vi "Consumer.vi"(8 "error in (no error)":errorcluster, 9 "Data":variant, 10 "Case ID":string, 11 "Kasli Wrapper in":refnum<class "Kasli Wrapper 2.0.lvclass">) -> (0 "error out":errorcluster, 3 "Kasli Wrapper out":refnum<class "Kasli Wrapper 2.0.lvclass">)   [LabVIEW 2020, in "Kasli Wrapper 2.0.lvlib" / "Kasli Wrapper 2.0.lvclass"]
uses:
  Kasli Wrapper 2.0.lvclass
  C:/Users/marco/Documents/GitHub_Lab/TALOS/talos/Ancestor/Ancestor/Ancestor.lvclass
  C:/Users/marco/Documents/GitHub_Lab/TALOS/talos/Father of all uServices/Father of all uServices/Father of all uServices.lvclass
  Kasli Wrapper 2.0 Consumer Case Selector.ctl
  Ancestor/Ancestor/Ancestor.lvclass/Ancestor.ctl
  Father of all uServices/Father of all uServices/Father of all uServices.lvclass/Father of all uServices.ctl
  Run Utilities/TypeDefs/Messages/Submit Message.ctl
  Run Utilities/TypeDefs/DAQ Control.ctl
  Run Utilities/Run Instance/Run Instance.lvclass
  Father of all uServices/Father of all uServices Messages/Consumer Msg/Consumer Msg.lvclass/Consumer Msg.ctl
  Kasli Wrapper 2.0.lvclass/Kasli Wrapper 2.0.ctl
  Std Selector.ctl
  Guardian/Guardian Messages/Message to uService Msg/Message to uService Msg.lvclass/Message to uService Msg.ctl
  Guardian/Guardian/Requests.ctl
  Guardian/Guardian Messages/Requests from uServices Msg/Requests from uServices Msg.lvclass/Requests from uServices Msg.ctl
  Classes/Log/Log.lvclass/Log.ctl
  Ancestor/Ancestor/Read ID.vi
  Guardian/Guardian Messages/Requests from uServices Msg/Send Requests from uServices.vi
  Guardian/Guardian Messages/Message to uService Msg/Send Message to uService.vi
  Classes/Log/Write.vi
  FGV/Error Memory/Get Error Description.vi
  Support VIs/Get PC name.vi
  Support VIs/Get Class Name.vi
  Support VIs/Date n Time.vi
  FGV/Error Memory/Error Memory Core.vi
  <vilib>/AdvancedString/Delimited String to 1D String Array.vi
  Support VIs/Circus Root Path.vi
  FGV/Error Memory/Error Crt Lvl checker.vi
  FGV/Error Memory/Error Memory Core.vi/40c8088d-b597-4017-91af-faa98e00292e.vi
  FGV/Error Memory/Error Memory Core.vi/d4a3ab98-063c-4e44-b43d-fbdcfe6c2be2.vi
  Father of all uServices/Father of all uServices/Father of all uServices.lvclass
  C:/Users/marco/Documents/GitHub_Lab/TALOS/builds/Actor Framework PPL/Actor Framework.lvlibp/1abvi3w/vi.lib/ActorFramework/Actor/Actor.lvclass
  Support VIs/Global Memory.vi
  <vilib>/Utility/LVClass/Get LV Class Name.vi
  Support VIs/Is in Packed Library.vi
  Support VIs/TALOS Root path.vi
  Support VIs/Read CSV worksheet.vi
  Support VIs/Global Constants.vi
  <vilib>/Utility/error.llb/General Error Handler.vi
  Support VIs/Error Log.vi
  builds/Actor Framework PPL/Actor Framework.lvlibp/1abvi3w/vi.lib/ActorFramework/Actor/Read Self Enqueuer.vi
  <userlib>/_OpenG.lib/lvdata/lvdata.llb/Get Strings from Enum__ogtk.vi
  builds/Actor Framework PPL/Actor Framework.lvlibp/1abvi3w/vi.lib/ActorFramework/Message Enqueuer/Enqueue.vi
  Father of all uServices/Father of all uServices/Children Methods/Get GUI Item Value - String.vi
  Father of all uServices/Father of all uServices/Multiline string updater.vi
  builds/Actor Framework PPL/Actor Framework.lvlibp/1abvi3w/vi.lib/ActorFramework/Actor/Read Caller Enqueuer.vi
  Classes/Log/Rotate.vi
  Ancestor/Ancestor/Ancestor.lvclass
  <vilib>/Comparison/Equal/Equal Functor/Equal Functor.lvclass
  Father of all uServices/Father of all uServices Messages/Consumer Msg/Consumer Msg.lvclass
  <vilib>/regexp/Match Regular Expression.xnode
  Guardian/Guardian Messages/Requests from uServices Msg/Requests from uServices Msg.lvclass
  Guardian/Guardian Messages/Message to uService Msg/Message to uService Msg.lvclass
  Run Utilities/Run Utilities.lvlib
  TALOS.lvlib
  Classes/Log/Log.lvclass
  Guardian/Guardian/Guardian.lvclass
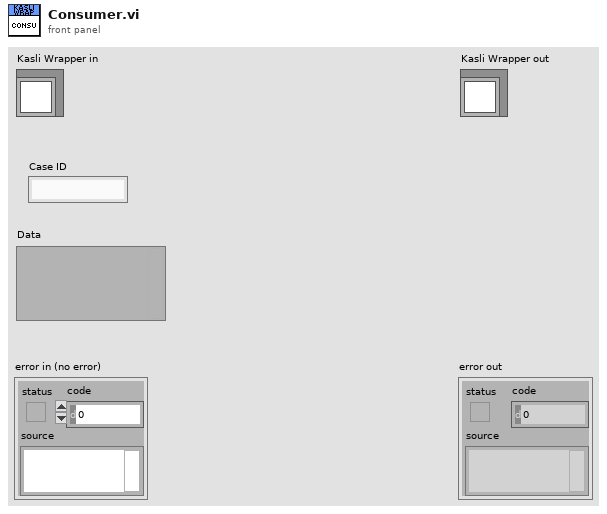
[diagram p1: front panel]
types:
  T1 = typedef "Kasli Wrapper 2.0.lvlib/Kasli Wrapper 2.0.lvclass/Kasli Wrapper 2.0 Consumer Case Selector.ctl" = enum16{"Init", "Submit Script", "Restart Master", "Master StdOut", "Master StdErr", "Client StdOut", "Client StdErr", "Start Logging", "Stop Logging", "Terminate Script", "Close", "Master ProcessExit"}
  T2 = cluster{"Font Name:":string, "Size":i16, "Strikeout?":bool, "Italic?":bool, "Underline?":bool, "Outline?":bool, "Shadow?":bool, "Bold?":bool}
  T3 = enum16{"User-specified Font", "Application Font", "System Font", "Dialog Font"}
  T4 = typedef "TALOS.lvlib/Run Utilities.lvlib/Submit Message.ctl" = cluster{"DAQ Control":T5, "Run Instance":refnum<class "Run Instance.lvclass">}
  T5 = typedef "TALOS.lvlib/Run Utilities.lvlib/DAQ Control.ctl" = enum16{"On", "Off", "External"}
  T6 = typedef "Kasli Wrapper 2.0.lvlib/Kasli Wrapper 2.0.lvclass/Std Selector.ctl" = enum16{"StdOut", "StdErr"}
  T7 = typedef "TALOS.lvlib/Guardian.lvlib/Guardian.lvclass/Requests.ctl" = enum16{"Ready to Launch", "Start RUN", "Stop RUN", "Update DAQ Params", "Update Error Listbox", "Update Run Status", "Update Kasli Log", "Run Stopped with Errors", "Switch uS View"}
  T8 = cluster{"left":i16, "top":i16, "right":i16, "bottom":i16}
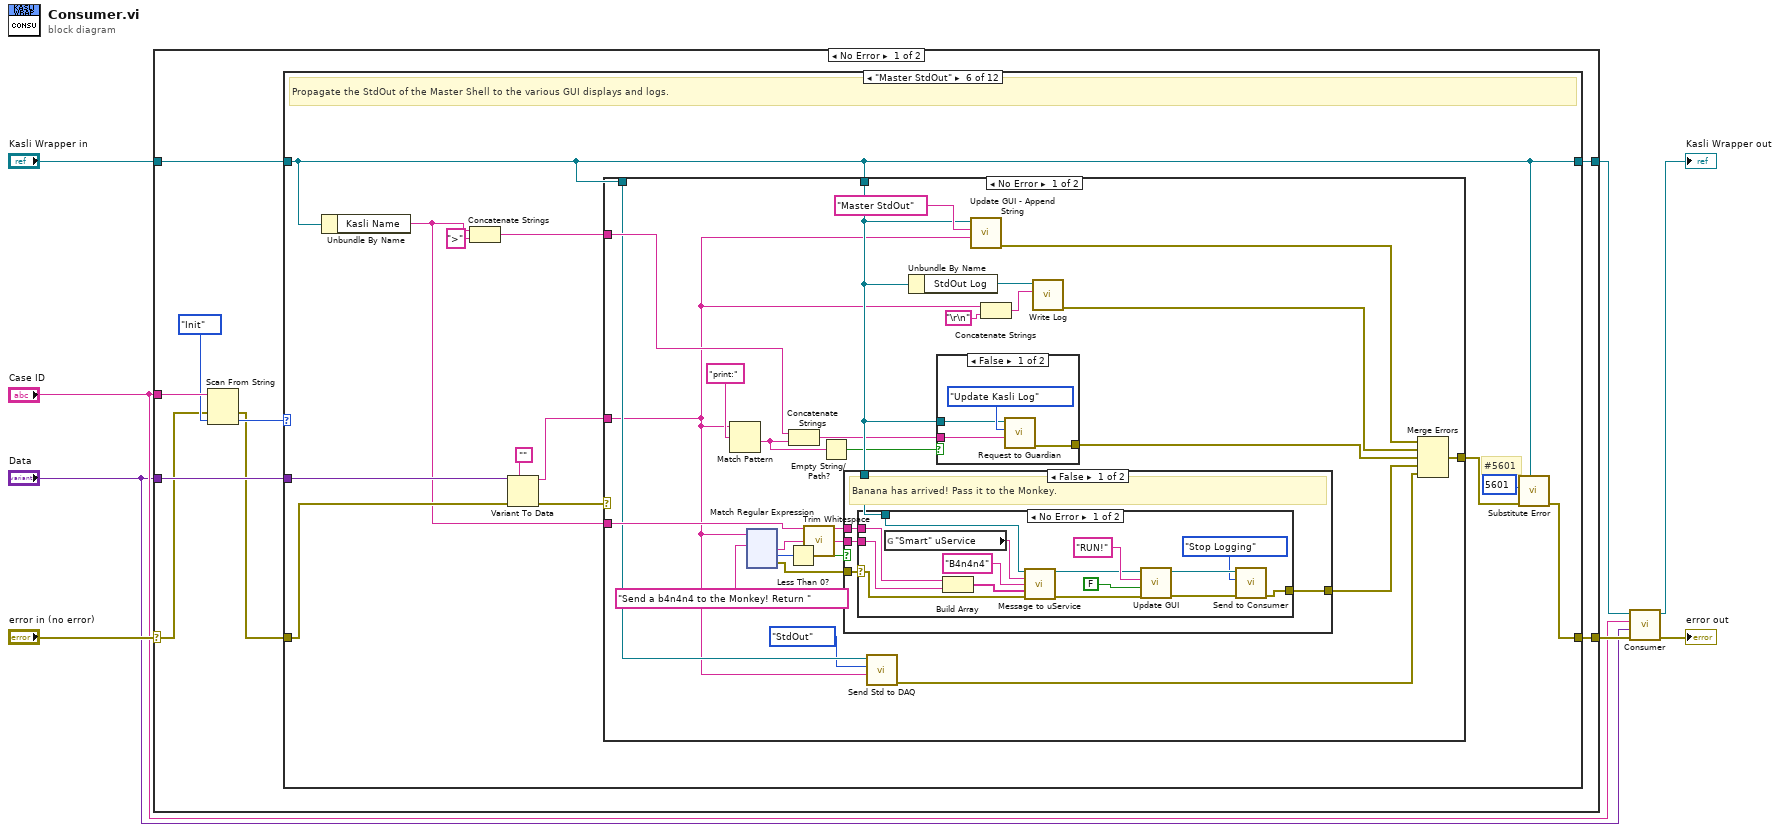
[diagram p0: block diagram]
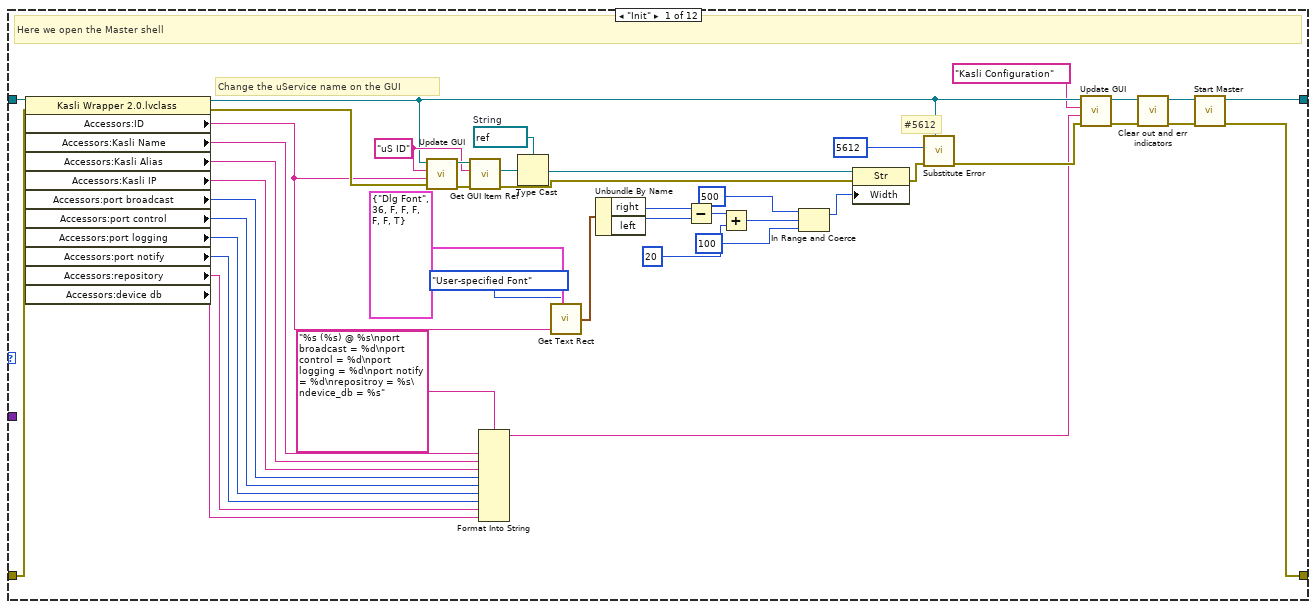
[diagram p2: hidden frame]
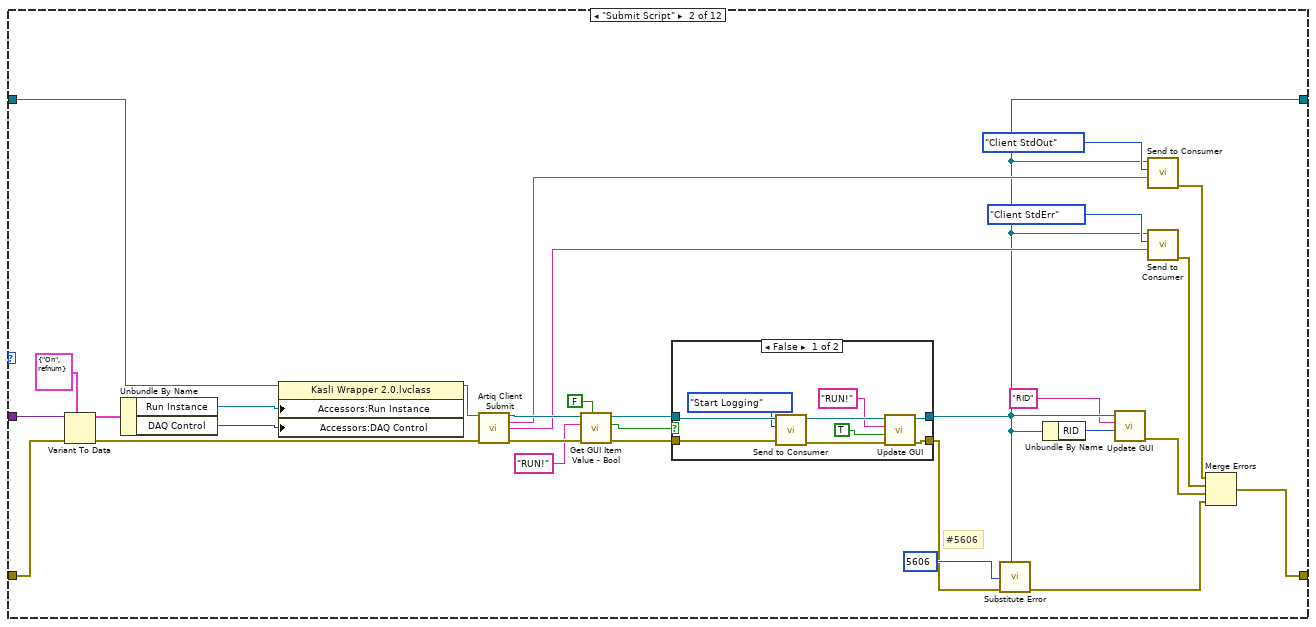
[diagram p3: hidden frame]
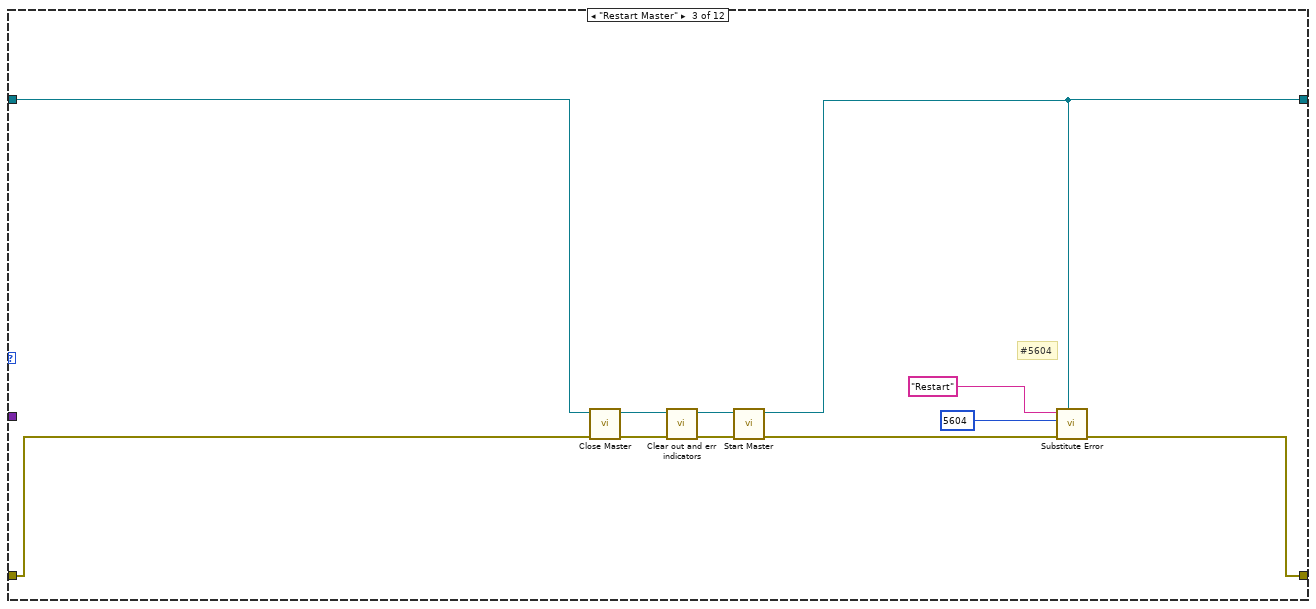
[diagram p5: hidden frame]
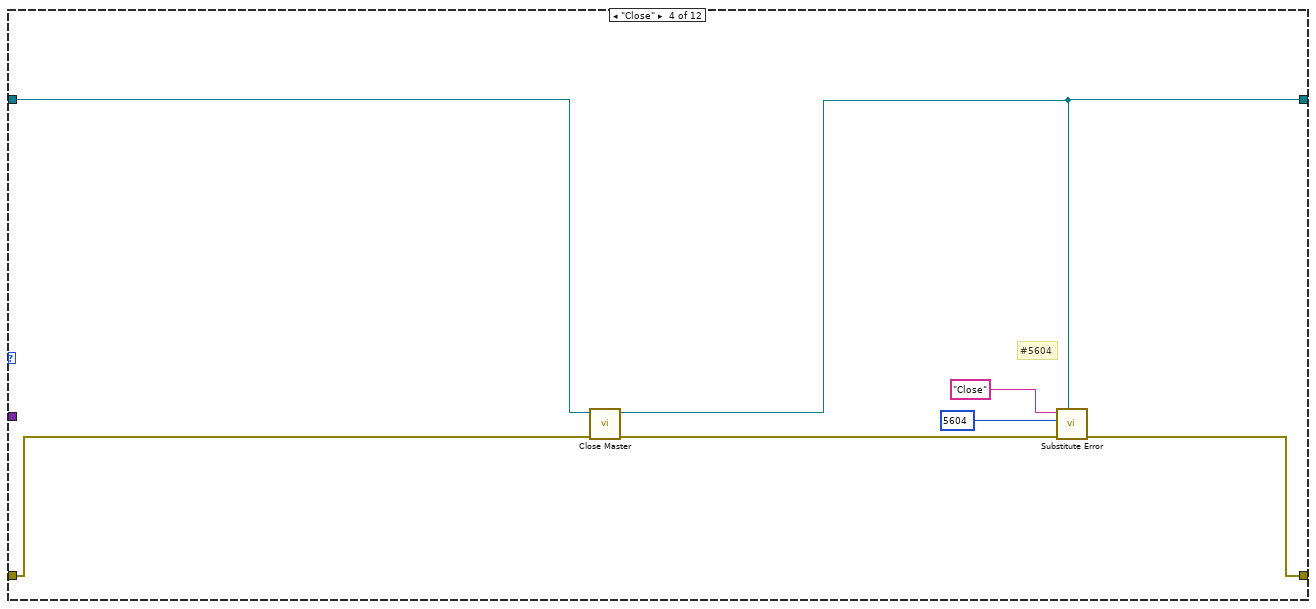
[diagram p6: hidden frame]
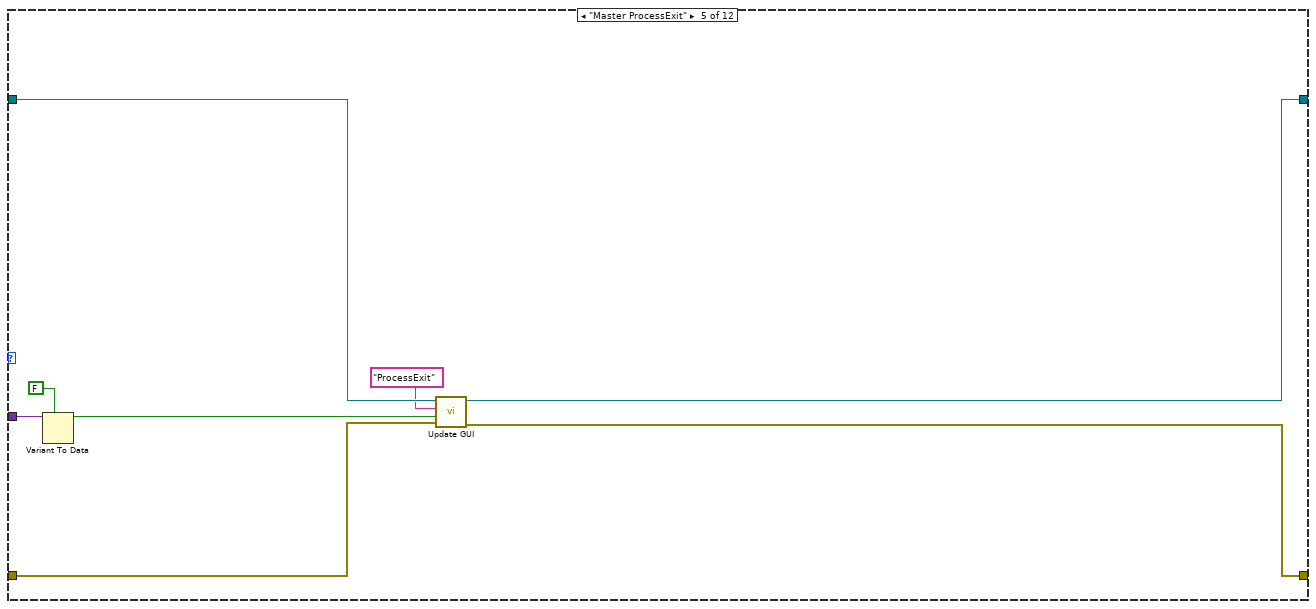
[diagram p7: hidden frame]
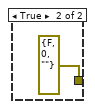
[diagram p8: hidden frame]
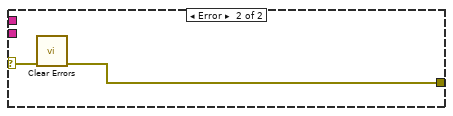
[diagram p9: hidden frame]
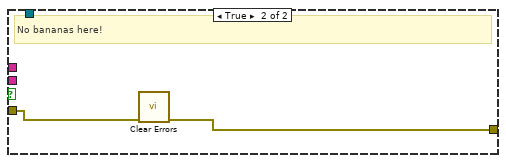
[diagram p10: hidden frame]
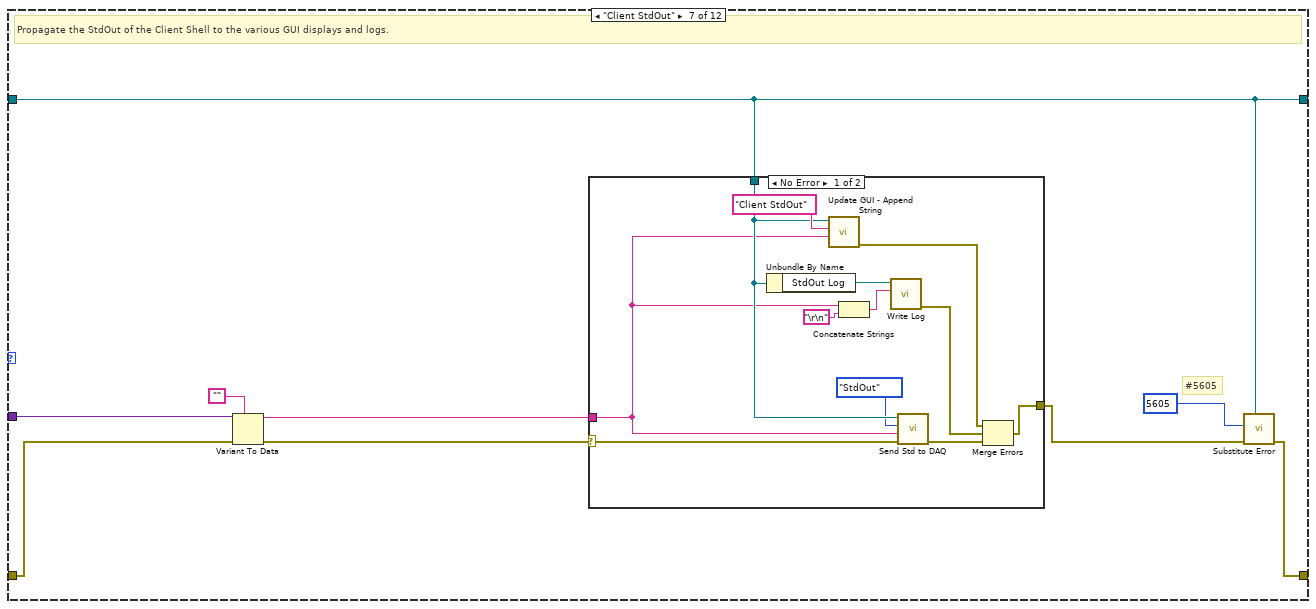
[diagram p12: hidden frame]
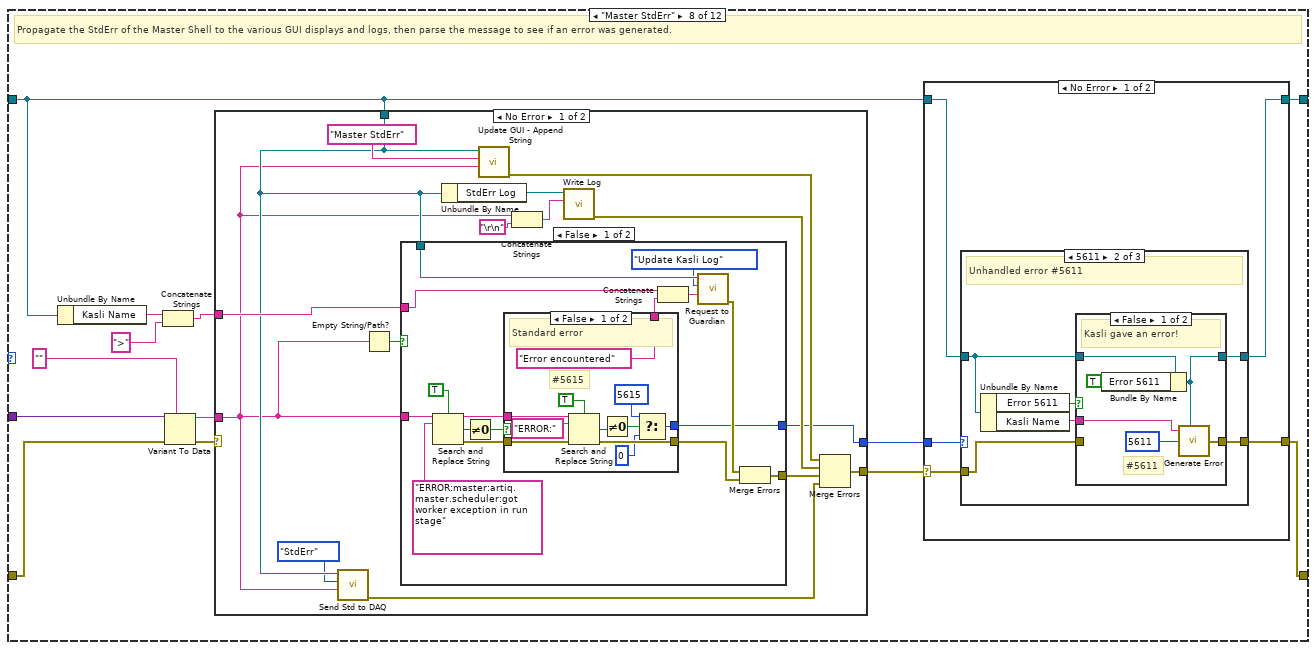
[diagram p14: hidden frame]
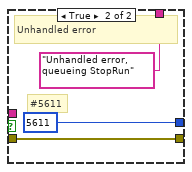
[diagram p15: hidden frame]
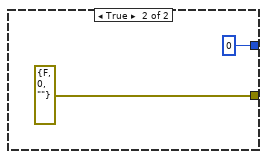
[diagram p16: hidden frame]
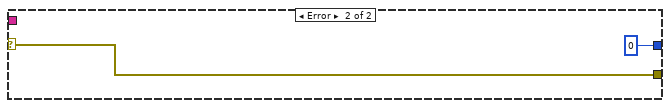
[diagram p17: hidden frame]
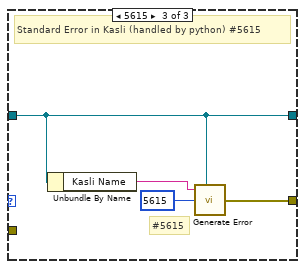
[diagram p20: hidden frame]
diagram:
  n1 = case shown="No Error" "error in (no error)" {
    selector: "error in (no error)" -> [w10 w537]
    tunnel: [w16 w538] -> w3
    tunnel: "Kasli Wrapper in" -> [w17 w538]
    tunnel: [w14 w537] -> w6
    tunnel: "Case ID" -> [w13 _]
    tunnel: "Data" -> [w15 _]
    frame No Error {
      n2 = Scan From String(input string=w13, error in=w10, default 1=Kasli_Wrapper_2.0_Consumer_Case_Selector."Init" ("Consumer Case Selector")) -> (error out=w9:errorcluster, output 1=w11:T1)  [unwired: 2 in, 2 out]
      n3 = case shown="\"Master StdOut\"" w11 {
        tunnel: w17 -> [w38 w75 w110 w117 w126 w129 w312 w334 w424 w482 w493 w509]
        tunnel: [w61 w64 w109 w116 w122 w129 w312 w333 w424 w484 w495 w501] -> w16
        tunnel: w15 -> [_ w90 _ _ w128 w140 w319 w345 w432 _ _ w508]
        tunnel: [w39 w86 w113 w120 w123 w133 w313 w340 w427 w483 w497 w502] -> w14
        tunnel: w9 -> [w37 w89 w112 w119 w124 w138 w317 w343 w430 w464 w492 w510]
        frame "Init" {
          w44 = refnum<vi> refnum  # String
          w43 = "uS ID" ("GUI Item Name")
          # "Change the uService name on the GUI"
          # "#5612"
          # "Here we open the Master shell"
          n4 = property class="Kasli Wrapper 2.0.lvclass"(reference=w38, error in=w37) -> (reference out=w25:refnum<class "Kasli Wrapper 2.0.lvclass">, error out=w53:errorcluster, "Accessors:ID"=w41:string, "Accessors:Kasli Name"=w26:string, "Accessors:Kasli Alias"=w35:string, "Accessors:Kasli IP"=w33:string, "Accessors:port broadcast"=w32:u32, "Accessors:port control"=w31:u32, "Accessors:port logging"=w30:u32, "Accessors:port notify"=w29:u32, "Accessors:repository"=w28:string, "Accessors:device db"=w27:string)
          n5 = call "Update GUI.vi"("error in (no error)"=w53, "Data"=w41, "GUI Item Name"=w43, "uService Template in"=w25) -> ("error out"=w51:errorcluster, "uService Template out"=w50:refnum<class "Kasli Wrapper 2.0.lvclass">)  [unwired: 6 in]
          n6 = call "Get GUI Item Ref.vi"("error in (no error)"=w51, "FP Item Name"=w43, "uService Template in"=w50) -> ("error out"=w55:errorcluster, "Ctl Refnum"=w52:refnum<vi>)  [unwired: 6 in, 1 out]
          n7 = Format Into String(format string="%s (%s) @ %s\nport broadcast = %d\nport control = %d\nport logging = %d\nport notify = %d\nrepositroy = %s\ndevice_db = %s", w26, w35, w33, w32, w31, w30, w29, w28, w27) -> (resulting string=w23:string)  [unwired: 2 in, 1 out]
          n8 = Type Cast(type=w44, x=w52) -> (*(type *) &x=w54:refnum<vi>)
          n9 = call <vilib>:"Get Text Rect.vi"("desired font(Application)"=T3."User-specified Font", "text"=w41, "[user-specified font]"=T2 {"Font Name:"="Dlg Font", "Size"=36, "Strikeout?"=FALSE, "Italic?"=FALSE, "Underline?"=FALSE, "Outline?"=FALSE, "Shadow?"=FALSE, "Bold?"=TRUE}) -> ("rect"=w42:T8)  [unwired: 6 in]
          n10 = Unbundle By Name(w42) -> ("right"=w56:i16, "left"=w57:i16)
          n11 = Subtract(x=w56, y=w57) -> (x-y=w58:i16)
          n12 = Add(x=w58, y=i16 20) -> (x+y=w59:i16)
          n13 = In Range and Coerce(upper limit=i16 500, x=w59, lower limit=i16 100) -> (coerced(x)=w60:i16)  [unwired: 1 out]
          n14 = property class="Str"(reference=w54, error in=w55, "Width"=w60) -> (error out=w36:errorcluster)  [unwired: 1 out]
          n15 = call "Substitute Error.vi"("LabVIEW Object"=w25, "error in (no error)"=w36, "Error Code"=5612) -> ("error out"=w24:errorcluster)  [unwired: 8 in]
          n16 = call "Update GUI.vi"("error in (no error)"=w24, "Data"=w23, "GUI Item Name"="Kasli Configuration", "uService Template in"=w25) -> ("error out"=w20:errorcluster, "uService Template out"=w21:refnum<class "Kasli Wrapper 2.0.lvclass">)  [unwired: 6 in]
          n17 = call-dynamic "Clear out and err indicators.vi"("error in (no error)"=w20, "Kasli Wrapper 2.0 in"=w21) -> ("error out"=w18:errorcluster, "Kasli Wrapper 2.0 out"=w19:refnum<class "Kasli Wrapper 2.0.lvclass">)  [unwired: 8 in]
          n18 = call "Start Master.vi"("error in (no error)"=w18, "Kasli Wrapper in"=w19) -> ("error out"=w39:errorcluster, "Kasli Wrapper out"=w61:refnum<class "Kasli Wrapper 2.0.lvclass">)  [unwired: 8 in]
        }
        frame "Submit Script" {
          # "#5606"
          n19 = Variant To Data(error in=w89, type=T4 {"DAQ Control"=enum."On", "Run Instance"=refnum} ("Submit Msg"), Variant=w90) -> (data=w78:T4, error out=w88:errorcluster)
          n20 = Unbundle By Name(w78) -> ("Run Instance"=w74:refnum<class "Run Instance.lvclass">, "DAQ Control"=w73:T5)
          n21 = property class="Kasli Wrapper 2.0.lvclass"(reference=w75, "Accessors:Run Instance"=w74, "Accessors:DAQ Control"=w73) -> (reference out=w72:refnum<class "Kasli Wrapper 2.0.lvclass">)  [unwired: 1 in, 1 out]
          n22 = call "Artiq Client Submit.vi"("Kasli Wrapper in"=w72, "error in (no error)"=w88) -> ("Kasli Wrapper out"=w91:refnum<class "Kasli Wrapper 2.0.lvclass">, "standard output"=w83:string, "standard error"=w82:string, "error out"=w71:errorcluster)  [unwired: 9 in, 1 out]
          n23 = call "Get GUI Item Value - Bool.vi"("Default"=FALSE, "error in (no error)"=w71, "FP Item Name"="RUN!", "uService Template in"=w91) -> ("error out"=w67:errorcluster, "Value"=w66:bool, "uService Template out"=w68:refnum<class "Kasli Wrapper 2.0.lvclass">)  [unwired: 5 in]
          n24 = case shown="False" w66 {
            tunnel: w68 -> [w99 w102]
            tunnel: w67 -> [w98 w101]
            tunnel: [w93 w102] -> w64
            tunnel: [w92 w101] -> w65
            frame False {
              n25 = call "Send to Consumer.vi"("error in (no error)"=w98, "Case ID"=Kasli_Wrapper_2.0_Consumer_Case_Selector."Start Logging" ("Consumer Case Selector"), "uService Template in"=w99) -> ("error out"=w94:errorcluster, "uService Template out"=w100:refnum<class "Kasli Wrapper 2.0.lvclass">)  [unwired: 7 in]
              n26 = call "Update GUI.vi"("error in (no error)"=w94, "Data"=TRUE ("Go?"), "GUI Item Name"="RUN!", "uService Template in"=w100) -> ("error out"=w92:errorcluster, "uService Template out"=w93:refnum<class "Kasli Wrapper 2.0.lvclass">)  [unwired: 6 in]
            }
            frame True {
            }
          }
          n27 = call "Substitute Error.vi"("LabVIEW Object"=w64, "error in (no error)"=w65, "Error Code"=5606) -> ("error out"=w62:errorcluster)  [unwired: 8 in]
          n28 = Unbundle By Name(w64) -> ("RID"=w76:u32)
          n29 = call "Update GUI.vi"("Data"=w76, "GUI Item Name"="RID", "uService Template in"=w64) -> ("error out"=w77:errorcluster)  [unwired: 7 in, 1 out]
          n30 = call "Send to Consumer.vi"("Data"=w83, "Case ID"=Kasli_Wrapper_2.0_Consumer_Case_Selector."Client StdOut" ("Consumer Case Selector"), "uService Template in"=w64) -> ("error out"=w80:errorcluster)  [unwired: 7 in, 1 out]
          n31 = call "Send to Consumer.vi"("Data"=w82, "Case ID"=Kasli_Wrapper_2.0_Consumer_Case_Selector."Client StdErr" ("Consumer Case Selector"), "uService Template in"=w64) -> ("error out"=w81:errorcluster)  [unwired: 7 in, 1 out]
          n32 = Merge Errors(w80, w81, w77, w62) -> (w86:errorcluster)
        }
        frame "Restart Master" {
          # "#5604"
          n33 = call "Close Master.vi"("error in (no error)"=w112, "Kasli Wrapper 2 in"=w110) -> ("error out"=w105:errorcluster, "Kasli Wrapper 2 out"=w106:refnum<class "Kasli Wrapper 2.0.lvclass">)  [unwired: 8 in]
          n34 = call-dynamic "Clear out and err indicators.vi"("error in (no error)"=w105, "Kasli Wrapper 2.0 in"=w106) -> ("error out"=w103:errorcluster, "Kasli Wrapper 2.0 out"=w104:refnum<class "Kasli Wrapper 2.0.lvclass">)  [unwired: 8 in]
          n35 = call "Start Master.vi"("error in (no error)"=w103, "Kasli Wrapper in"=w104) -> ("error out"=w108:errorcluster, "Kasli Wrapper out"=w109:refnum<class "Kasli Wrapper 2.0.lvclass">)  [unwired: 8 in]
          n36 = call "Substitute Error.vi"("LabVIEW Object"=w109, "error in (no error)"=w108, "Error Code"=5604, "Optional String"="Restart") -> ("error out"=w113:errorcluster)  [unwired: 7 in]
        }
        frame "Close" {
          # "#5604"
          n37 = call "Close Master.vi"("error in (no error)"=w119, "Kasli Wrapper 2 in"=w117) -> ("error out"=w115:errorcluster, "Kasli Wrapper 2 out"=w116:refnum<class "Kasli Wrapper 2.0.lvclass">)  [unwired: 8 in]
          n38 = call "Substitute Error.vi"("LabVIEW Object"=w116, "error in (no error)"=w115, "Error Code"=5604, "Optional String"="Close") -> ("error out"=w120:errorcluster)  [unwired: 7 in]
        }
        frame "Master ProcessExit" {
          n39 = Variant To Data(type=FALSE, Variant=w128) -> (data=w125:bool)  [unwired: 1 in, 1 out]
          n40 = call "Update GUI.vi"("error in (no error)"=w124, "Data"=w125, "GUI Item Name"="ProcessExit", "uService Template in"=w126) -> ("error out"=w123:errorcluster, "uService Template out"=w122:refnum<class "Kasli Wrapper 2.0.lvclass">)  [unwired: 6 in]
        }
        frame "Master StdOut" {
          # "#5601"
          # "Propagate the StdOut of the Master Shell to the various GUI displays and logs."
          n41 = Unbundle By Name(w129) -> ("Kasli Name"=w130:string)
          n42 = Concatenate Strings(w130, ">" ("string")) -> (w131:string)
          n43 = Variant To Data(error in=w138, type="", Variant=w140) -> (data=w137:string, error out=w136:errorcluster)
          n44 = case shown="No Error" w136 {
            selector: w136 -> [_ w310]
            tunnel: w129 -> [w153 _]
            tunnel: w137 -> [w142 _]
            tunnel: [w166 w310] -> w134
            tunnel: w131 -> [w145 _]
            tunnel: w130 -> [w146 _]
            tunnel: w129 -> [w144 _]
            frame No Error {
              n45 = Match Pattern(string=w142, regular expression="print:") -> (after substring=w147:string)  [unwired: 1 in, 3 out]
              n46 = xnode "Match Regular Expression"("input string"=w142, "regular expression"="Send a b4n4n4 to the Monkey! Return " ("search string")) -> ("after match"=w155:string, "offset past match"=w157:i32, "error out"=w154:errorcluster)  [unwired: 4 in, 2 out]
              n47 = Less Than 0?(x=w157) -> (x < 0?=w156:bool)
              n48 = Concatenate Strings(w145, w147) -> (w149:string)
              n49 = call <vilib>:"Trim Whitespace.vi"("string"=w155) -> ("trimmed string"=w151:string)  [unwired: 1 in]
              n50 = Empty String/Path?(string/path=w147) -> (empty?=w148:bool)
              n51 = case shown="False" w156 {
                tunnel: w151 -> [w289 _]
                tunnel: w154 -> [w288 w309]
                tunnel: w153 -> [w290 _]
                tunnel: [w287 w308] -> w152
                tunnel: w146 -> [w286 _]
                frame False {
                  # "Banana has arrived! Pass it to the Monkey."
                  n52 = case shown="No Error" w288 {
                    selector: w288 -> [w301 w307]
                    tunnel: w290 -> [w305 _]
                    tunnel: w289 -> [w303 _]
                    tunnel: [w293 w306] -> w287
                    tunnel: w286 -> [w300 _]
                    frame No Error {
                      n53 = global read "Global Constants.vi" "\"Smart\" uService"() -> (w299:string)
                      n54 = Build Array(w300, w303) -> (w302:string[])
                      n55 = call "Message to uService.vi"("Father of all uServices in"=w305, "uService ID"=w299, "Message"="B4n4n4", "Data"=w302, "error in (no error)"=w301) -> ("Father of all uServices out"=w295:refnum<class "Kasli Wrapper 2.0.lvclass">, "error out"=w296:errorcluster)  [unwired: 9 in]
                      n56 = call "Update GUI.vi"("error in (no error)"=w296, "Data"=FALSE ("Go?"), "GUI Item Name"="RUN!", "uService Template in"=w295) -> ("error out"=w294:errorcluster, "uService Template out"=w292:refnum<class "Kasli Wrapper 2.0.lvclass">)  [unwired: 6 in]
                      n57 = call "Send to Consumer.vi"("error in (no error)"=w294, "Case ID"=Kasli_Wrapper_2.0_Consumer_Case_Selector."Stop Logging" ("Consumer Case Selector"), "uService Template in"=w292) -> ("error out"=w293:errorcluster)  [unwired: 7 in, 1 out]
                    }
                    frame Error {
                      n58 = call <vilib>:"Clear Errors.vi"("error in (no error)"=w307) -> ("error out"=w306:errorcluster)  [unwired: 5 in, 1 out]
                    }
                  }
                }
                frame True {
                  # "No bananas here!"
                  n59 = call <vilib>:"Clear Errors.vi"("error in (no error)"=w309) -> ("error out"=w308:errorcluster)  [unwired: 5 in, 1 out]
                }
              }
              n60 = call-dynamic "Send Std to DAQ.vi"("New Message"=w142, "Std Selector"=Std_Selector."StdOut", "Kasli Wrapper 2.0 in"=w144) -> ("error out"=w141:errorcluster)  [unwired: 7 in, 1 out]
              n61 = Unbundle By Name(w153) -> ("StdOut Log"=w165:refnum<class "Log.lvclass">)
              n62 = case shown="False" w148 {
                tunnel: [w170 errorcluster {"status"=FALSE, "code"=0, "source"=""} ("error out")] -> w150
                tunnel: w153 -> [w168 _]
                tunnel: w149 -> [w167 _]
                frame False {
                  n63 = call "Request to Guardian.vi"("Data"=w167, "Requests"=Requests."Update Kasli Log", "Father of all uServices in"=w168) -> ("error out"=w170:errorcluster)  [unwired: 7 in, 1 out]
                }
                frame True {
                }
              }
              n64 = call "Update GUI - Append String.vi"("String"=w142, "GUI Item Name"="Master StdOut", "Father of all uServices in"=w153) -> ("error out"=w160:errorcluster)  [unwired: 7 in, 1 out]
              n65 = Concatenate Strings(w142, "\r\n") -> (w164:string)
              n66 = call "Write Log.vi"("Text"=w164, "Log in"=w165) -> ("error out"=w162:errorcluster)  [unwired: 8 in, 1 out]
              n67 = Merge Errors(w160, w162, w150, w152, w141) -> (w166:errorcluster)
            }
            frame Error {
            }
          }
          n68 = call "Substitute Error.vi"("LabVIEW Object"=w129, "error in (no error)"=w134, "Error Code"=5601) -> ("error out"=w133:errorcluster)  [unwired: 8 in]
        }
        frame "Client StdOut" {
          # "#5605"
          # "Propagate the StdOut of the Client Shell to the various GUI displays and logs."
          n69 = Variant To Data(error in=w317, type="", Variant=w319) -> (data=w316:string, error out=w315:errorcluster)
          n70 = case shown="No Error" w315 {
            selector: w315 -> [w321 w332]
            tunnel: w312 -> [w324 _]
            tunnel: w316 -> [w323 _]
            tunnel: [w331 w332] -> w311
            frame No Error {
              n71 = Unbundle By Name(w324) -> ("StdOut Log"=w330:refnum<class "Log.lvclass">)
              n72 = call "Update GUI - Append String.vi"("String"=w323, "GUI Item Name"="Client StdOut", "Father of all uServices in"=w324) -> ("error out"=w325:errorcluster)  [unwired: 7 in, 1 out]
              n73 = Concatenate Strings(w323, "\r\n") -> (w329:string)
              n74 = call "Write Log.vi"("Text"=w329, "Log in"=w330) -> ("error out"=w327:errorcluster)  [unwired: 8 in, 1 out]
              n75 = call-dynamic "Send Std to DAQ.vi"("error in (no error)"=w321, "New Message"=w323, "Std Selector"=Std_Selector."StdOut", "Kasli Wrapper 2.0 in"=w324) -> ("error out"=w322:errorcluster)  [unwired: 6 in, 1 out]
              n76 = Merge Errors(w325, w327, w322) -> (w331:errorcluster)
            }
            frame Error {
            }
          }
          n77 = call "Substitute Error.vi"("LabVIEW Object"=w312, "error in (no error)"=w311, "Error Code"=5605) -> ("error out"=w313:errorcluster)  [unwired: 8 in]
        }
        frame "Master StdErr" {
          # "Propagate the StdErr of the Master Shell to the various GUI displays and logs, then parse the message to see if an error was generated."
          n78 = Unbundle By Name(w334) -> ("Kasli Name"=w337:string)
          n79 = Concatenate Strings(w337, ">" ("string")) -> (w335:string)
          n80 = Variant To Data(error in=w343, type="", Variant=w345) -> (data=w342:string, error out=w341:errorcluster)
          n81 = case shown="No Error" w341 {
            selector: w341 -> [_ w394]
            tunnel: w334 -> [w351 _]
            tunnel: w342 -> [w348 _]
            tunnel: [w346 0 ("number of replacements")] -> w339
            tunnel: [w360 w394] -> w338
            tunnel: w335 -> [w353 _]
            frame No Error {
              n82 = call-dynamic "Send Std to DAQ.vi"("New Message"=w348, "Std Selector"=Std_Selector."StdErr", "Kasli Wrapper 2.0 in"=w351) -> ("error out"=w349:errorcluster)  [unwired: 7 in, 1 out]
              n83 = Empty String/Path?(string/path=w348) -> (empty?=w352:bool)
              n84 = case shown="False" w352 {
                tunnel: w351 -> [w376 _]
                tunnel: w353 -> [w362 _]
                tunnel: w348 -> [w371 _]
                tunnel: [w373 errorcluster {"status"=FALSE, "code"=0, "source"=""} ("error out")] -> w347
                tunnel: [w364 0 ("Error Code")] -> w346
                frame False {
                  n85 = Search and Replace String(case sensitive?=TRUE ("ignore case? (F)"), input string=w371, search string="ERROR:master:artiq.master.scheduler:got worker exception in run stage") -> (result string=w365:string, number of replacements=w369:i32, error out=w367:errorcluster)  [unwired: 5 in, 1 out]
                  n86 = Not Equal To 0?(x=w369) -> (x != 0?=w368:bool)
                  n87 = case shown="False" w368 {
                    tunnel: w367 -> [w387 w390]
                    tunnel: [w386 w390] -> w366
                    tunnel: w365 -> [w385 _]
                    tunnel: [w378 5611 ("Error Code")] -> w364
                    tunnel: ["Error encountered" "Unhandled error, queueing StopRun"] -> w363
                    frame False {
                      # "#5615"
                      # "Standard error"
                      n88 = Search and Replace String(case sensitive?=TRUE ("ignore case? (F)"), input string=w385, search string="ERROR:", error in=w387) -> (number of replacements=w382:i32, error out=w386:errorcluster)  [unwired: 4 in, 2 out]
                      n89 = Not Equal To 0?(x=w382) -> (x != 0?=w381:bool)
                      n90 = Select(t=5615, s=w381, f=0 ("Error Code")) -> (s? t:f=w378:i32)
                    }
                    frame True {
                      # "#5611"
                      # "Unhandled error"
                    }
                  }
                  n91 = Concatenate Strings(w362, w363) -> (w361:string)
                  n92 = call "Request to Guardian.vi"("Data"=w361, "Requests"=Requests."Update Kasli Log", "Father of all uServices in"=w376) -> ("error out"=w374:errorcluster)  [unwired: 7 in, 1 out]
                  n93 = Merge Errors(w374, w366) -> (w373:errorcluster)
                }
                frame True {
                }
              }
              n94 = Unbundle By Name(w351) -> ("StdErr Log"=w358:refnum<class "Log.lvclass">)
              n95 = call "Update GUI - Append String.vi"("String"=w348, "GUI Item Name"="Master StdErr", "Father of all uServices in"=w351) -> ("error out"=w354:errorcluster)  [unwired: 7 in, 1 out]
              n96 = Concatenate Strings(w348, "\r\n") -> (w359:string)
              n97 = call "Write Log.vi"("Text"=w359, "Log in"=w358) -> ("error out"=w356:errorcluster)  [unwired: 8 in, 1 out]
              n98 = Merge Errors(w354, w356, w347, w349) -> (w360:errorcluster)
            }
            frame Error {
            }
          }
          n99 = case shown="No Error" w338 {
            selector: w338 -> [w396 w422]
            tunnel: w339 -> [w395 _]
            tunnel: [w397 w421] -> w340
            tunnel: w334 -> [w399 w420]
            tunnel: [w398 w420] -> w333
            frame No Error {
              n100 = case shown="5611" w395 {
                tunnel: w399 -> [w401 w405 w417]
                tunnel: [w401 w407 w417] -> w398
                tunnel: [w400 w406 w419] -> w397
                tunnel: w396 -> [w400 w404 _]
                frame 0, Default {
                  # "All good, this is just a warning"
                }
                frame 5611 {
                  # "Unhandled error #5611"
                  n101 = Unbundle By Name(w405) -> ("Error 5611"=w402:bool, "Kasli Name"=w403:string)
                  n102 = case shown="False" w402 {
                    tunnel: w405 -> [w410 w415]
                    tunnel: [w409 w415] -> w407
                    tunnel: [w411 w414] -> w406
                    tunnel: w404 -> [_ w414]
                    tunnel: w403 -> [w408 _]
                    frame False {
                      # "#5611"
                      # "Kasli gave an error!"
                      n103 = Bundle By Name(cluster=w410, "Error 5611"=TRUE ("Error 6666")) -> (w409:refnum<class "Kasli Wrapper 2.0.lvclass">)
                      n104 = call "Generate Error.vi"("Optional String"=w408, "Class"=w409, "Error Code"=5611) -> ("error out"=w411:errorcluster)  [unwired: 4 in]
                    }
                    frame True {
                      # "Everything's good!"
                    }
                  }
                }
                frame 5615 {
                  # "#5615"
                  # "Standard Error in Kasli (handled by python) #5615"
                  n105 = Unbundle By Name(w417) -> ("Kasli Name"=w416:string)
                  n106 = call "Generate Error.vi"("Optional String"=w416, "Class"=w417, "Error Code"=5615) -> ("error out"=w419:errorcluster)  [unwired: 4 in]
                }
              }
            }
            frame Error {
              # "#5602"
              n107 = call "Substitute Error.vi"("LabVIEW Object"=w420, "error in (no error)"=w422, "Error Code"=5602) -> ("error out"=w421:errorcluster)  [unwired: 8 in]
            }
          }
        }
        frame "Client StdErr" {
          # "Propagate the StdErr of the Client Shell to the various GUI displays and logs, then parse the message to see if an error was generated."
          n108 = Variant To Data(error in=w430, type="", Variant=w432) -> (data=w429:string, error out=w428:errorcluster)
          n109 = case shown="No Error" w428 {
            selector: w428 -> [w448 w450]
            tunnel: w424 -> [w435 _]
            tunnel: w429 -> [w436 _]
            tunnel: [w447 0 ("number of replacements")] -> w426
            tunnel: [w445 w450] -> w425
            frame No Error {
              n110 = Unbundle By Name(w435) -> ("StdErr Log"=w443:refnum<class "Log.lvclass">)
              n111 = call-dynamic "Send Std to DAQ.vi"("New Message"=w436, "Std Selector"=Std_Selector."StdErr", "Kasli Wrapper 2.0 in"=w435) -> ("error out"=w433:errorcluster)  [unwired: 7 in, 1 out]
              n112 = Concatenate Strings(w436, "\r\n") -> (w444:string)
              n113 = Search and Replace String(case sensitive?=TRUE ("ignore case? (F)"), input string=w436, search string="error", error in=w448) -> (number of replacements=w447:i32, error out=w446:errorcluster)  [unwired: 4 in, 2 out]
              n114 = call "Update GUI - Append String.vi"("String"=w436, "GUI Item Name"="Client StdErr", "Father of all uServices in"=w435) -> ("error out"=w440:errorcluster)  [unwired: 7 in, 1 out]
              n115 = call "Write Log.vi"("Text"=w444, "Log in"=w443) -> ("error out"=w437:errorcluster)  [unwired: 8 in, 1 out]
              n116 = Merge Errors(w440, w437, w446, w433) -> (w445:errorcluster)
            }
            frame Error {
            }
          }
          n117 = case shown="No Error" w425 {
            selector: w425 -> [w453 w462]
            tunnel: w426 -> [w455 _]
            tunnel: [w452 w461] -> w427
            tunnel: w424 -> [w451 w460]
            frame No Error {
              n118 = Not Equal To 0?(x=w455) -> (x != 0?=w454:bool)
              n119 = case shown="True" w454 {
                tunnel: w453 -> [w456 _]
                tunnel: [w456 w458] -> w452
                tunnel: w451 -> [_ w457]
                frame False {
                  # "Everything's good!"
                }
                frame True {
                  # "#5614"
                  # "Kasli gave an error!"
                  n120 = call "Generate Error.vi"("Class"=w457, "Error Code"=5614) -> ("error out"=w458:errorcluster)  [unwired: 5 in]
                }
              }
            }
            frame Error {
              # "#5606"
              n121 = call "Substitute Error.vi"("LabVIEW Object"=w460, "error in (no error)"=w462, "Error Code"=5606) -> ("error out"=w461:errorcluster)  [unwired: 8 in]
            }
          }
        }
        frame "Start Logging" {
          w467 = "_" ("t")
          w469 = "Kasli" ("t")
          # "#5618"
          # "#5617"
          n122 = property class="Kasli Wrapper 2.0.lvclass"(reference=w482) -> (reference out=w475:refnum<class "Kasli Wrapper 2.0.lvclass">, "Accessors:Kasli Name"=w468:string)  [unwired: 1 in, 1 out]
          n123 = Empty String/Path?(string/path=w468) -> (empty?=w470:bool)
          n124 = Concatenate Strings(w467, w468, w467) -> (w466:string)
          n125 = Select(t=w467, s=w470, f=w466) -> (s? t:f=w465:string)
          n126 = Concatenate Strings(w469, w465, "StdOut" ("Name")) -> (w473:string)
          n127 = Concatenate Strings(w469, w465, "StdErr" ("Name")) -> (w471:string)
          n128 = call "New Log.vi"("Specific Error Code"=5617, "Name"=w473) -> ("error out"=w477:errorcluster, "Log out"=w479:refnum<class "Log.lvclass">)  [unwired: 8 in]
          n129 = call "New Log.vi"("Specific Error Code"=5618, "Name"=w471) -> ("error out"=w476:errorcluster, "Log out"=w478:refnum<class "Log.lvclass">)  [unwired: 8 in]
          n130 = Bundle By Name(cluster=w475, "StdOut Log"=w479, "StdErr Log"=w478) -> (w484:refnum<class "Kasli Wrapper 2.0.lvclass">)
          n131 = Merge Errors(w477, w476, w464) -> (w483:errorcluster)
        }
        frame "Stop Logging" {
          w487 = "end of transmissions"
          # "Run Stopped: immediately send the log files to the DAQ before it closes!"
          n132 = call-dynamic "Send Std to DAQ.vi"("Just send!"=TRUE, "New Message"=w487, "Std Selector"=Std_Selector."StdErr", "Kasli Wrapper 2.0 in"=w493) -> ("error out"=w485:errorcluster)  [unwired: 6 in, 1 out]
          n133 = call-dynamic "Send Std to DAQ.vi"("Just send!"=TRUE, "New Message"=w487, "Std Selector"=Std_Selector."StdOut", "Kasli Wrapper 2.0 in"=w493) -> ("error out"=w486:errorcluster)  [unwired: 6 in, 1 out]
          n134 = Merge Errors(w486, w485) -> (w496:errorcluster)
          n135 = Bundle By Name(cluster=w493, "Batman"="") -> (w495:refnum<class "Kasli Wrapper 2.0.lvclass">)
          n136 = Merge Errors(w496, w492) -> (w497:errorcluster)
        }
        frame "Terminate Script" {
          w499 = FALSE  # Gracefully
          # "Calls artiq-client delete to stop the script and then submits the same script with the _TerminationRequested=TRUE"
          n137 = Variant To Data(type=w499, Variant=w508) -> (data=w500:bool, error out=w512:errorcluster)  [unwired: 1 in]
          n138 = Select(t=w499, s=w512, f=w500) -> (s? t:f=w498:bool)
          n139 = call "Artiq Client Delete.vi"("Kasli Wrapper in"=w509, "error in (no error)"=w510) -> ("Kasli Wrapper out"=w511:refnum<class "Kasli Wrapper 2.0.lvclass">, "standard output"=w505:string, "standard error"=w504:string, "error out"=w503:errorcluster)  [unwired: 9 in, 1 out]
          n140 = call "Send to Consumer.vi"("Data"=w505, "Case ID"=Kasli_Wrapper_2.0_Consumer_Case_Selector."Client StdOut" ("Consumer Case Selector"), "uService Template in"=w511) -> ()  [unwired: 7 in, 2 out]
          n141 = call "Send to Consumer.vi"("Data"=w504, "Case ID"=Kasli_Wrapper_2.0_Consumer_Case_Selector."Client StdErr" ("Consumer Case Selector"), "uService Template in"=w511) -> ()  [unwired: 7 in, 2 out]
          n142 = case shown="True" w498 {
            tunnel: w511 -> [w520 w536]
            tunnel: w503 -> [w519 w535]
            tunnel: [w513 w533] -> w502
            tunnel: [w514 w522] -> w501
            frame False {
              # "Not gracefully, just stop the script and finish logging"
              n143 = call "Send to Consumer.vi"("error in (no error)"=w519, "Case ID"=Kasli_Wrapper_2.0_Consumer_Case_Selector."Stop Logging" ("Consumer Case Selector"), "uService Template in"=w520) -> ("error out"=w515:errorcluster, "uService Template out"=w521:refnum<class "Kasli Wrapper 2.0.lvclass">)  [unwired: 7 in]
              n144 = call "Update GUI.vi"("error in (no error)"=w515, "Data"=FALSE ("Go?"), "GUI Item Name"="RUN!", "uService Template in"=w521) -> ("error out"=w513:errorcluster, "uService Template out"=w514:refnum<class "Kasli Wrapper 2.0.lvclass">)  [unwired: 6 in]
            }
            frame True {
              # "submit the script"
              # "Add the termination flag"
              # "Gracefully terminating script means that the _TerminationRequested=true is added to the parameters and script is run again. This flag makes script exit at the beginning and go straight to the closure function"
              n145 = Unbundle By Name(w536) -> ("DAQ Control"=w525:T5, "Run Instance"=w531:refnum<class "Run Instance.lvclass">)
              n146 = Build Array("_TerminationRequested", "true" ("element")) -> (w528:string[])
              n147 = Build Array(w528) -> (w527:string[][])
              n148 = call-dynamic "Update Parameters.vi"("error in (no error)"=w535, "Parameters"=w527, "Run Instance in"=w531) -> ("error out"=w534:errorcluster, "Run Instance out"=w524:refnum<class "Run Instance.lvclass">)  [unwired: 6 in, 1 out]
              n149 = Bundle(cluster=T4 {"DAQ Control"=enum."On", "Run Instance"=refnum} ("Submit Msg"), "DAQ Control"=w525, "Run Instance"=w524) -> (w523:T4)
              n150 = call "Send to Consumer.vi"("error in (no error)"=w534, "Data"=w523, "Case ID"=Kasli_Wrapper_2.0_Consumer_Case_Selector."Submit Script" ("Consumer Case Selector"), "uService Template in"=w536) -> ("error out"=w533:errorcluster, "uService Template out"=w522:refnum<class "Kasli Wrapper 2.0.lvclass">)  [unwired: 6 in]
            }
          }
        }
      }
    }
    frame Error {
    }
  }
  n151 = call-parent "Consumer.vi"("error in (no error)"=w6, "Data"="Data", "Case ID"="Case ID", "uService Template in"=w3) -> ("error out"=→"error out":errorcluster, "uService Template out"=→"Kasli Wrapper out":refnum<class "Kasli Wrapper 2.0.lvclass">)  [unwired: 6 in]
